vi "Handle Last Ack Core.vi"(4 "error in (no error)":errorcluster, 6 "Last Ack":refnum<class "Last Ack.lvclass">, 7 "IModel in":refnum<class "IModel.lvclass">) -> (0 "error out":errorcluster, 3 "IModel out":refnum<class "IModel.lvclass">)   [LabVIEW 2020, in "IModel.lvlib" / "IModel.lvclass"]
uses:
  <vilib>/gpm_packages/@cs/mva-core/Source/IModel/IModel/IModel.lvclass
  <vilib>/ActorFramework/LastAck/Last Ack.lvclass
  C:/Program Files/National Instruments/LabVIEW 2020/vi.lib/gpm_packages/@cs/mva-core/Source/IObserver/IObserver/IObserver.lvclass
  C:/Program Files/National Instruments/LabVIEW 2020/vi.lib/ActorFramework/Actor/Actor.lvclass
  <vilib>/ActorFramework/LastAck/Last Ack.lvclass/Last Ack.ctl
  <vilib>/ActorFramework/Message/Message.lvclass
  <vilib>/gpm_packages/@cs/mva-core/Source/IObserver/IObserver/IObserver.lvclass/IObserver.ctl
  <vilib>/gpm_packages/@cs/event-logger/Source/Composed Log/LoggerReference/LoggerReference.lvclass/LoggerReference.ctl
  <vilib>/gpm_packages/@cs/mva-core/Source/IModel/IModel/IModel.lvclass/IModel.ctl
  <vilib>/ActorFramework/Actor/Actor.lvclass/Actor.ctl
  <vilib>/ActorFramework/Message Enqueuer/Message Enqueuer.lvclass/Message Enqueuer.ctl
  <vilib>/gpm_packages/@cs/event-logger/Source/Composed Log/LoggerReference/Log Event.vi
  <vilib>/ActorFramework/Actor/Read Self Enqueuer.vi
  <vilib>/ActorFramework/Message Enqueuer/Enqueue.vi
  <vilib>/gpm_packages/@cs/event-logger/Source/Composed Log/LoggerReference/Log.vi
  <vilib>/gpm_packages/@cs/event-logger/Source/Composed Log/LoggerReference/Get Valid Event Time.vi
  <vilib>/ActorFramework/Message Enqueuer/Init from Existing Queue.vi
  <vilib>/gpm_packages/@cs/event-logger/Source/Composed Log/LoggerReference/Remove Stale Logs.vi
  <vilib>/ActorFramework/Message Priority Queue/Priority Enqueue.vi
  <vilib>/ActorFramework/Message Enqueuer/Message Enqueuer.lvclass
  <vilib>/gpm_packages/@cs/mva-core/Source/IObserver/IObserver/IObserver.lvclass
  <vilib>/ActorFramework/Actor/Actor.lvclass
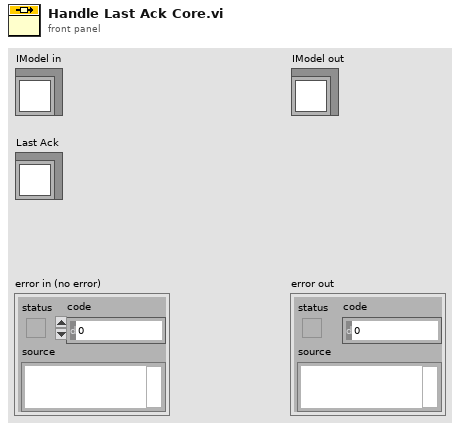
[diagram p1: front panel]
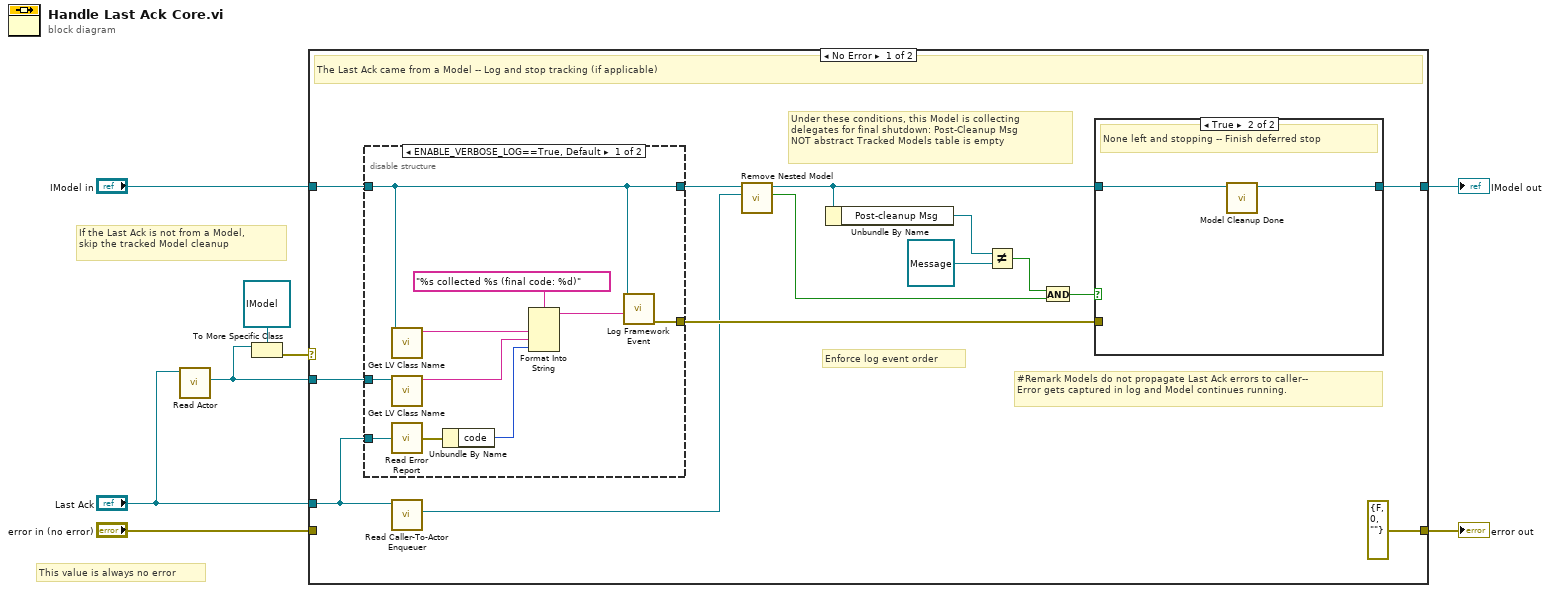
[diagram p0: block diagram]
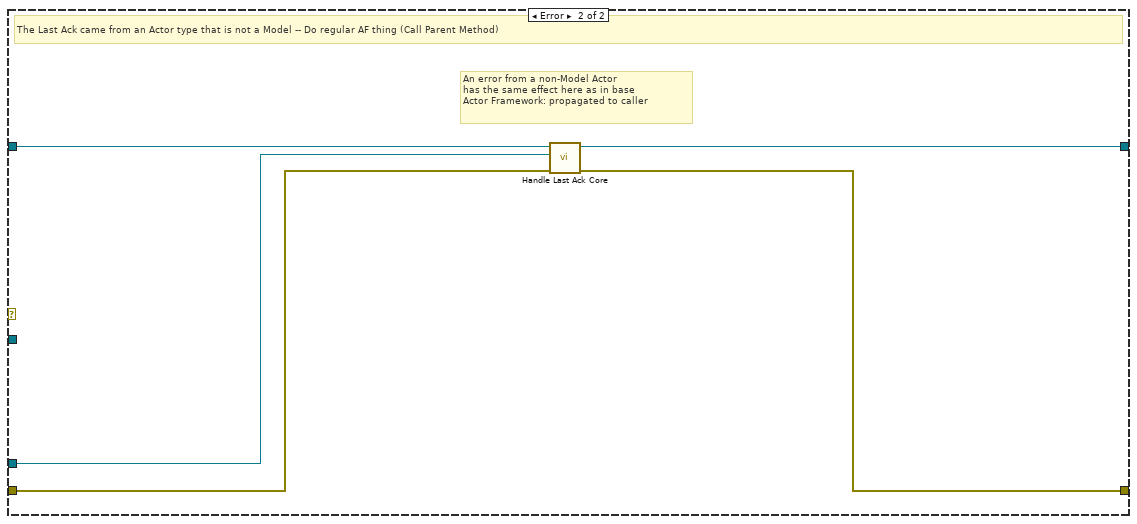
[diagram p4: hidden frame]
diagram:
  # "If the Last Ack is not from a Model,\nskip the tracked Model cleanup"
  # "This value is always no error"
  n1 = call <vilib>:"Read Actor.vi"("Last Ack"="Last Ack") -> ("Actor"=w1:refnum<class "Actor.lvclass">)  [unwired: 10 in]
  n2 = To More Specific Class(target class=refnum<class "IModel.lvclass"> refnum ("IModel.lvlib:IModel.lvclass"), reference=w1) -> (error out=w3:errorcluster)  [unwired: 1 in, 1 out]
  n3 = case shown="No Error" w3 {
    tunnel: "Last Ack" -> [w17 w37]
    tunnel: [w22 w40] -> w7
    tunnel: "IModel in" -> [w21 w41]
    tunnel: [errorcluster {"status"=FALSE, "code"=0, "source"=""} ("error IO") w38] -> w5
    tunnel: w1 -> [w18 _]
    tunnel: "error in (no error)" -> [_ w39]
    frame No Error {
      # "Enforce log event order"
      # "Under these conditions, this Model is collecting\ndelegates for final shutdown: Post-Cleanup Msg\nNOT abstract Tracked Models table is empty"
      # "#Remark Models do not propagate Last Ack errors to caller--\nError gets captured in log and Model continues running."
      # "The Last Ack came from a Model -- Log and stop tracking (if applicable)"
      n4 = disable-structure shown="ENABLE_VERBOSE_LOG==True, Default" {
        disable-tunnel: w17 -> [w32 _]
        disable-tunnel: [w29 _] -> w10
        disable-tunnel: w21 -> [w28 w33]
        disable-tunnel: [w28 w33] -> w19
        disable-tunnel: w18 -> [w24 _]
        frame condition #0 (active) {
          # "Log Last Ack event"
          n5 = call <vilib>:"Get LV Class Name.vi"("object"=w28) -> ("class name"=w31:string)  [unwired: 9 in, 1 out]
          n6 = call <vilib>:"Get LV Class Name.vi"("object"=w24) -> ("class name"=w23:string)  [unwired: 9 in, 1 out]
          n7 = call <vilib>:"Read Error Report.vi"("Last Ack"=w32) -> ("error report"=w27:errorcluster)
          n8 = Unbundle By Name(w27) -> ("code"=w25:i32)
          n9 = Format Into String(format string="%s collected %s (final code: %d)", w31, w23, w25) -> (resulting string=w30:string)  [unwired: 2 in, 1 out]
          n10 = call <vilib>:"Log Framework Event.vi"("Data To Log"=w30, "IObserver in"=w28) -> ("error out"=w29:errorcluster)  [unwired: 9 in]
        }
        frame condition #1 {
          # "Remove all logging from this method at compile time"
        }
      }
      n11 = call <vilib>:"Read Caller-To-Actor Enqueuer.vi"("Last Ack"=w17) -> ("Caller-to-Actor Enqueuer"=w9:refnum<class "Message Enqueuer.lvclass">)  [unwired: 10 in]
      n12 = call <vilib>:"Remove Nested Model.vi"("Nested Model Enqueuer"=w9, "IModel in"=w19) -> ("None Remaining?"=w12:bool, "IModel out"=w14:refnum<class "IModel.lvclass">)  [unwired: 8 in]
      n13 = Unbundle By Name(w14) -> ("Post-cleanup Msg"=w13:refnum<class "Message.lvclass">)
      n14 = Not Equal?(x=w13, y=refnum<class "Message.lvclass"> refnum) -> (x != y?=w15:bool)
      n15 = And(x=w15, y=w12) -> (x .and. y?=w11:bool)
      n16 = case shown="True" w11 {
        tunnel: w14 -> [w34 w35]
        tunnel: [w34 w36] -> w22
        tunnel: w10 -> [_ _]
        frame False {
          # "Keep waiting for last acks"
        }
        frame True {
          # "None left and stopping -- Finish deferred stop"
          n17 = call <vilib>:"Model Cleanup Done.vi"("IModel in"=w35) -> ("IModel out"=w36:refnum<class "IModel.lvclass">)  [unwired: 10 in]
        }
      }
    }
    frame Error {
      # "An error from a non-Model Actor\nhas the same effect here as in base\nActor Framework: propagated to caller"
      # "The Last Ack came from an Actor type that is not a Model -- Do regular AF thing (Call Parent Method)"
      n18 = call-parent "Handle Last Ack Core.vi"("error in (no error)"=w39, "Last Ack"=w37, "Actor in"=w41) -> ("error out"=w38:errorcluster, "Actor out"=w40:refnum<class "IModel.lvclass">)  [unwired: 3 in]
    }
  }
  "IModel out" <- w7
  "error out" <- w5
